vi "Evaluate Start Trigger.vi"(8 "error in (no error)":errorcluster, 10 "Start Trigger Data":dbl[](array[numeric]), 11 "Triggered Log in":refnum<class "Triggered Log.lvclass">) -> (0 "error out":errorcluster, 3 "Triggered Log out":refnum<class "Triggered Log.lvclass">)   [LabVIEW 2012, in "Triggered Log.lvclass"]
doc: "Evaluate the trigger if the log is in the Waiting on Trigger state. Update the state according to the trigger. If the log transitions to the Triggered state, flush any pretrigger data and notify any registered listeners of the state change."
uses:
  Triggered Log.lvclass
  Triggered Log.lvclass/Triggered Log.ctl
  Triggered Log State.ctl
  Engine/Classes/Logs/Segmented Logs/Segmented Log/Segmented Log.lvclass/Segmented Log.ctl
  Shared/Classes/Log File Specifications/Log File Specification/Log File Specification.lvclass/Log File Specification.ctl
  Flush Buffer Data to File.vi
  On Triggered Log State Change.vi
  Flush Buffer Data.vi
  Engine/Classes/Logs/Segmented Logs/Segmented Log/Write Data to Log File Instance (Waveform).vi
  Engine/Classes/Logs/Segmented Logs/Segmented Log/Write Data to Log File Instance.vi
  Engine/Classes/Logs/Segmented Logs/Segmented Log/Check Close File.vi
  Engine/Classes/Logs/Segmented Logs/Segmented Log/Check Open File.vi
  Engine/Classes/Logs/Segmented Logs/Segmented Log/Close Log File Instance.vi
  Engine/Classes/Logs/Segmented Logs/Segmented Log/Open Log File Instance.vi
  Engine/Classes/Logs/Segmented Logs/Segmented Log/On Segmented Log Complete.vi
  Engine/Classes/Logs/Segmented Logs/Segmented Log/On File Close.vi
  Shared/Classes/Log File Specifications/Log File Specification/Open Log File.vi
  Shared/Classes/Log File Specifications/Log File Specification/Set Path Tag.vi
  Engine/Classes/Logs/Segmented Logs/Segmented Log/On File Open.vi
  Shared/Classes/Log File Specifications/Log File Specification/Set Filename Offset.vi
  Shared/Classes/Log File Specifications/Log File Specification/Build File Path.vi
  Shared/Classes/Log File Specifications/Log File Specification/Resolve File Conflicts.vi
  Engine/Classes/Triggers/Trigger/Initialize.vi
  Engine/Classes/Triggers/Trigger/Finalize.vi
  Shared/Classes/Log File Specifications/Log File Specification/Initialize Log File.vi
  <vilib>/Utility/libraryn.llb/Check if File or Folder Exists.vi
  <vilib>/Utility/error.llb/Error Cluster From Error Code.vi
  <vilib>/Utility/libraryn.llb/Get File Extension.vi
  <vilib>/Utility/libraryn.llb/Create Directory Recursive.vi
  Engine/Classes/Logs/Log Files/Log File/Write to Log File (Waveform).vi
  Engine/Classes/Logs/Segmented Logs/Segmented Log/Segment Log File.vi
  Engine/Classes/Logs/Log Files/Log File/Close Log File.vi
  Engine/Classes/Logs/Segmented Logs/Segmented Log/Make File Read-Only.vi
  Engine/Classes/Logs/Log Files/Log File/Write to Log File.vi
  Engine/Classes/Logs/Log Files/Log File/Log File.lvclass
  Engine/Classes/Triggers/Trigger/Trigger.lvclass
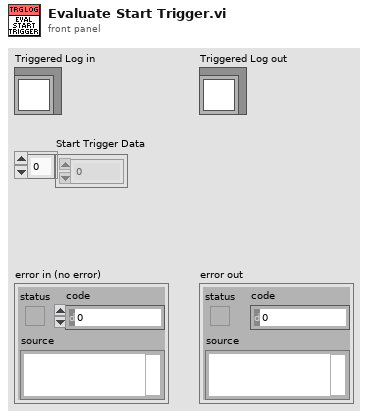
[diagram p1: front panel]
types:
  T1 = typedef "Triggered Log.lvclass/Triggered Log State.ctl" = enum16{"Waiting on Trigger", "Triggered", "Posttrigger", "Complete", "Idle", "Error"}
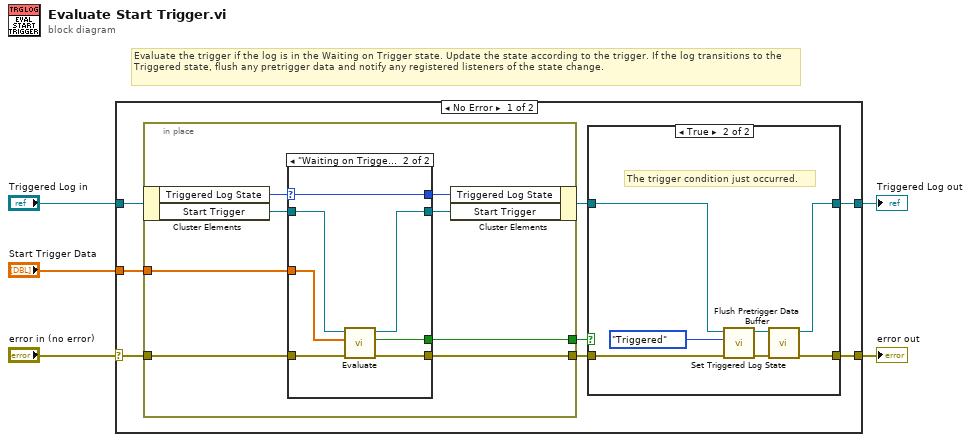
[diagram p0: block diagram]
diagram:
  # "Evaluate the trigger if the log is in the Waiting on Trigger state. Update the state according to the trigger. If the log transitions to the Triggered state, flush any pretrigger data and notify any registered listeners of the state change."
  n1 = case shown="No Error" "error in (no error)" {
    selector: "error in (no error)" -> [w12 w42]
    tunnel: [w6 w42] -> w5
    tunnel: [w8 w41] -> w4
    tunnel: "Start Trigger Data" -> [w11 _]
    tunnel: "Triggered Log in" -> [w13 w41]
    frame No Error {
      n2 = in-place {
        in-place-border: w12 -> [w30]
        in-place-border: w11 -> [w28]
        in-place-border: [w29] -> w10
        in-place-border: [w25] -> w9
        n3 = in-place-cluster #1(w13) -> ("Triggered Log State"=w26:T1, "Start Trigger"=w24:refnum<class "Trigger.lvclass">)
        n4 = case shown="\"Waiting on Trigger\"" w26 {
          selector: w26 -> [w33 w40]
          tunnel: w24 -> [w32 w39]
          tunnel: [w32 w35] -> w23
          tunnel: w30 -> [w31 w38]
          tunnel: [w31 w37] -> w29
          tunnel: w28 -> [_ w36]
          tunnel: [w33 w40] -> w27
          tunnel: [_ w34] -> w25
          frame Default {
            # "Only evaluate the trigger if the log is in the Waiting on Trigger state."
          }
          frame "Waiting on Trigger" {
            n5 = call "Evaluate.vi"("error in (no error)"=w38, "Trigger Data"=w36, "Trigger in"=w39) -> ("error out"=w37:errorcluster, "Trigger"=w34:bool, "Trigger out"=w35:refnum<class "Trigger.lvclass">)  [unwired: 6 in]
          }
        }
        n6 = in-place-cluster #1("Triggered Log State"=w27, "Start Trigger"=w23) -> (w7:refnum<class "Triggered Log.lvclass">)
      }
      n7 = case shown="True" w9 {
        tunnel: w10 -> [w14 w20]
        tunnel: [w15 w21] -> w8
        tunnel: w7 -> [w15 w19]
        tunnel: [w14 w22] -> w6
        frame False {
          # "The log has not changed state."
        }
        frame True {
          # "The trigger condition just occurred."
          n8 = call "Set Triggered Log State.vi"("error in (no error)"=w20, "Triggered Log State"=Triggered_Log_State."Triggered", "Triggered Log in"=w19) -> ("error out"=w16:errorcluster, "Triggered Log out"=w17:refnum<class "Triggered Log.lvclass">)  [unwired: 7 in]
          n9 = call "Flush Pretrigger Data Buffer.vi"("error in (no error)"=w16, "Triggered Log in"=w17) -> ("error out"=w22:errorcluster, "Triggered Log out"=w21:refnum<class "Triggered Log.lvclass">)  [unwired: 8 in]
        }
      }
    }
    frame Error {
    }
  }
  "error out" <- w5
  "Triggered Log out" <- w4
